vi "Update Controller.vi"(8 "error in":errorcluster, 11 "MultiController in":refnum<class "MultiController.lvclass">) -> (0 "error out":errorcluster, 3 "MultiController out":refnum<class "MultiController.lvclass">)   [LabVIEW 2012, in "MultiController.lvclass"]
doc: "Providing the correct RH and the setpoint, update the controller such that it provides the proper response."
uses:
  MultiController.lvclass
  MultiController.lvclass/MultiController.ctl
  Base/Humidity Control.lvclass/Humidity Control.ctl
  Base/Data Access/Read RHmeas.vi
  Base/Data Access/Read Tair.vi
  Base/Data Access/Read useTair.vi
  <vilib>/addons/control/pid/pid.llb/PID (DBL Array).vi
  <vilib>/addons/control/pid/pid.llb/PID Percentage to EGU (DBL Array).vi
  Base/Read RH.vi
  Base/Read PID.vi
  <vilib>/addons/control/pid/NI_PID_pid.lvlib
  General/Atmospheric/Atmospheric Library.lvlib
  Base/Humidity Control.lvclass
panel:
  out "Td (degC)":dbl[](array[numeric]) format="%.2f"
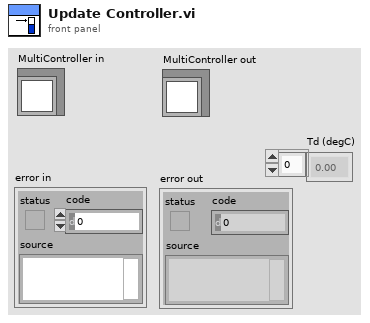
[diagram p1: front panel]
types:
  T1 = cluster{"proportional gain (Kc)":dbl, "integral time (Ti, min)":dbl, "derivative time (Td, min)":dbl}[]
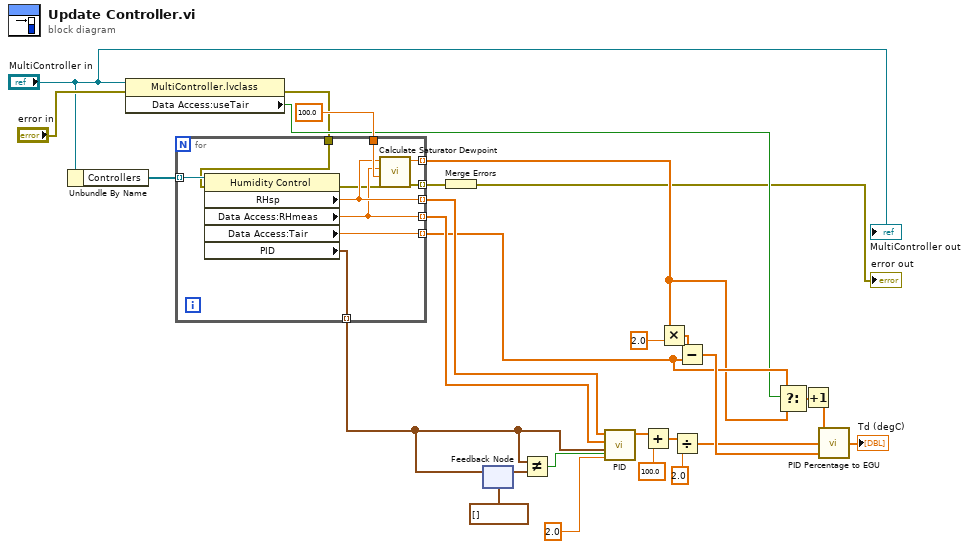
[diagram p0: block diagram]
diagram:
  n1 = Unbundle By Name("MultiController in") -> ("Controllers"=w13:refnum<class "Humidity Control.lvclass">[])
  n2 = property class="MultiController.lvclass"(reference="MultiController in", error in="error in") -> (error out=w3:errorcluster, "Data Access:useTair"=w5:bool)  [unwired: 1 out]
  n3 = for {
    tunnel: w13 -> [w38] mode=indexing
    tunnel: [w34] -> w12 mode=indexing
    tunnel: [w33] -> w11 mode=indexing
    tunnel: [w37] -> w10 mode=indexing
    tunnel: [w36] -> w9 mode=indexing
    tunnel: 100.0 ("RH_sat_out") -> [w35]
    tunnel: [w31] -> w6 mode=indexing
    tunnel: [w30] -> w7 mode=indexing
    tunnel: w3 -> [w29]
    n4 = property class="Humidity Control"(reference=w38, error in=w29) -> (error out=w32:errorcluster, "RHsp"=w34:dbl, "Data Access:RHmeas"=w33:dbl, "Data Access:Tair"=w37:dbl, "PID"=w36:cluster{"P":dbl, "I":dbl, "D":dbl})  [unwired: 1 out]
    n5 = call "Calculate Saturator Dewpoint.vi"("error in"=w32, "RH_sat_out"=w35, "Tair"=w33, "RH_tar"=w34) -> ("error out"=w31:errorcluster, "Td"=w30:dbl)  [unwired: 6 in]
  }
  n6 = Merge Errors(w6) -> (→"error out":errorcluster)
  n7 = feedback #1(T1 []) -> (w27:T1)
  n8 = feedback-in #1(w9) -> ()
  n9 = Not Equal?(x=w9, y=w27) -> (x != y?=w26:bool)
  n10 = call-poly <vilib>:"PID.vi"("reinitialize? (F)"=w26, "dt (s)"=2.0, "PID gains"=w9, "process variable"=w11, "setpoint"=w12) -> ("output"=w23:dbl[])  [unwired: 5 in, 1 out]
  n11 = Add(x=w23, y=100.0) -> (x+y=w21:dbl[])
  n12 = Multiply(x=w7, y=2.0) -> (x*y=w24:dbl[])
  n13 = Divide(x=w21, y=2.0) -> (x/y=w18:dbl[])
  n14 = Subtract(x=w24, y=w10) -> (x-y=w19:dbl[])
  n15 = Select(t=w10, s=w5, f=w7) -> (s? t:f=w15:dbl[])
  n16 = Increment(x=w15) -> (x+1=w14:dbl[])
  n17 = call-poly <vilib>:"PID Percentage to EGU.vi"("minimum (EGU)"=w19, "% span"=w18, "maximum (EGU)"=w14) -> ("output (EGU)"=→"Td (degC)":dbl[])  [unwired: 1 in]
  "MultiController out" <- "MultiController in"
